vi "Inspect Weight Fiducials.vi"(5 "Dispose Images?":bool, 6 "WorkTable Class in":refnum<class "WorkTable Class.lvclass">=refnum, 7 "Glue Pathways":T7 {"BBM Slot" items=["Slot 1", "Slot 2", "Slot 3", "Slot 4"]; "Weight Slot" items=["Slot 1", "Slot 2", "Slot 3", "Slot 4"]; "Glue Slot" items=["Slot 1", "Slot 2", "Slot 3", "Slot 4"]; "Stamp Slot" items=["Slot 1", "Slot 2", "Slot 3", "Slot 4"]; "HDI Slot" items=["Slot 1", "Slot 2", "Slot 3", "Slot 4"]}, 8 "error in":errorcluster, 9 "Console Log in":refnum<class "Console Log.lvclass">, 10 "Single Path in":T6, 11 "CameraTool in":refnum<class "CameraTool Class.lvclass">) -> (0 "error out":errorcluster, 1 "Console Log out":refnum<class "Console Log.lvclass">, 2 "Single Path out":T6, 3 "CameraTool out":refnum<class "CameraTool Class.lvclass">)   [LabVIEW 2017, in "Gluing Procedure.lvclass"]
uses:
  Gluing Procedure.lvclass
  Shared Components/Config Manager Class/Type Definitions/Named Position.ctl
  Shared Components/CameraTool Class/CameraTool Class.lvclass
  Application Utilities/Console Log/Console Log.lvclass
  UI typedefs/Glue Path.ctl
  Shared Components/WorkTable Class/WorkTable Class.lvclass
  Shared Components/Vec3d Class/Vec3d Class.lvclass
  <vilib>/vision/Image Controls.llb/IMAQ Image.ctl
  Shared Components/Utils/Type Definitions/Physical Image.ctl
  Shared Components/Utils/Type Definitions/Fiducial with Source.ctl
  Shared Components/Utils/Type Definitions/Fiducial Image.ctl
  Shared Components/Utils/Type Definitions/Part Fiducials.ctl
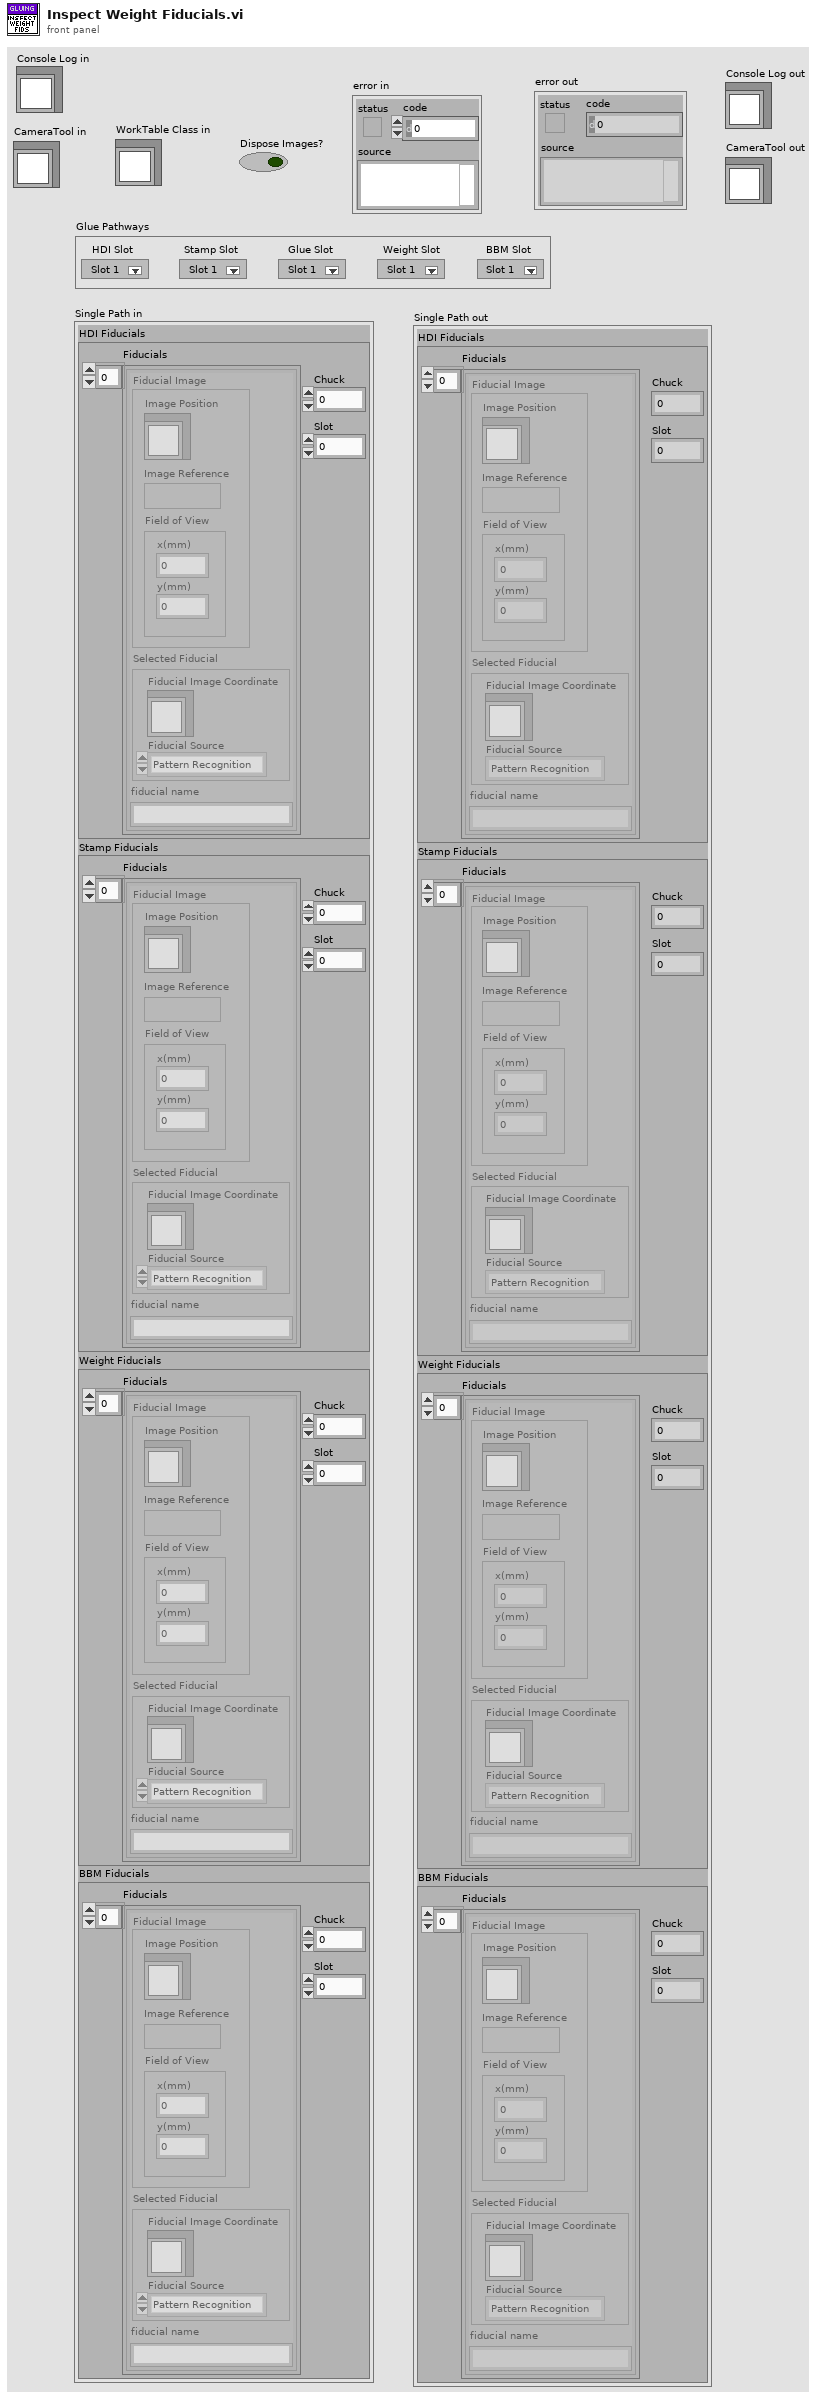
[diagram p1: front panel]
types:
  T1 = typedef "Part Fiducials.ctl" = cluster{"Fiducials":T2[], "Chuck":i32, "Slot":i32}
  T2 = typedef "Fiducial Image.ctl" = cluster{"Fiducial Image":T3, "Selected Fiducial":T5, "fiducial name":string}
  T3 = typedef "Physical Image.ctl" = cluster{"Image Position":refnum<class "Vec3d Class.lvclass">, "Image Reference":T4, "Field of View":cluster{"x(mm)":dbl, "y(mm)":dbl}}
  T4 = typedef "IMAQ Image.ctl" = refnum<image>
  T5 = typedef "Fiducial with Source.ctl" = cluster{"Fiducial Image Coordinate":refnum<class "Vec3d Class.lvclass">, "Fiducial Source":enum16{"Pattern Recognition", "User", "Error", "Default"}}
  T6 = cluster{"HDI Fiducials":T1, "Stamp Fiducials":T1, "Weight Fiducials":T1, "BBM Fiducials":T1}
  T7 = typedef "Glue Path.ctl" = cluster{"HDI Slot ":i32, "Stamp Slot":i32, "Glue Slot":i32, "Weight Slot":i32, "BBM Slot":i32}
  T8 = typedef "Named Position.ctl" = enum16{"home", "module_chuck_0", "module_chuck_1", "module_chuck_2", "module_chuck_3", "module_chuck_4", "glue_reservoir_chuck", "stamp_tool_chuck", "weight_tool_chuck", "needle_calibration", "needle_calibration_camera", "tool_rack_pos_0_in", "tool_rack_pos_0_out", "tool_rack_pos_1_in", "tool_rack_pos_1_out", "tool_rack_pos_2_in", "tool_rack_pos_2_out", "front_load_position", "grabber_start_pos", "between_chuck_0_and_1", "between_chuck_2_and_3"}
  T9 = typedef "Worktable_Weight.ctl" = cluster{"Weight State":enum16{"Empty", "Populated"}, "Weight Type":T10, "Location/Orientation":T11}
  T10 = typedef "Weight Type.ctl" = enum16{"Weight 1", "Weight 2", "Weight 3", "Weight 4", "Weight 5", "Weight 6", "Weight 7", "Weight 8", "Weight 9", "Weight 10", "Weight 11", "Weight 12", "Weight 13", "Weight 14", "Weight 15", "Weight 16"}
  T11 = typedef "Position_Orientation.ctl" = cluster{"Center":refnum<class "Vec3d Class.lvclass">, "Orientation":refnum<class "Orient3d Class.lvclass">}
  T12 = typedef "Part Type.ctl" = enum16{"BBM", "HDI", "BARE HDI", "GLUERESERVOIR", "STAMP_1", "STAMP_2", "STAMP_3", "STAMP_4", "STAMP_5", "STAMP_6", "STAMP_7", "STAMP_8", "WEIGHT_1", "WEIGHT_2", "WEIGHT_3", "WEIGHT_4", "WEIGHT_5", "WEIGHT_6", "WEIGHT_7", "WEIGHT_8", "WEIGHT_9", "WEIGHT_10", "WEIGHT_11", "WEIGHT_12", "WEIGHT_13", "WEIGHT_14", "WEIGHT_15", "WEIGHT_16", "PICKER_TOOL", "GRABER_TOOL", "TFPX_HDI_V2"}
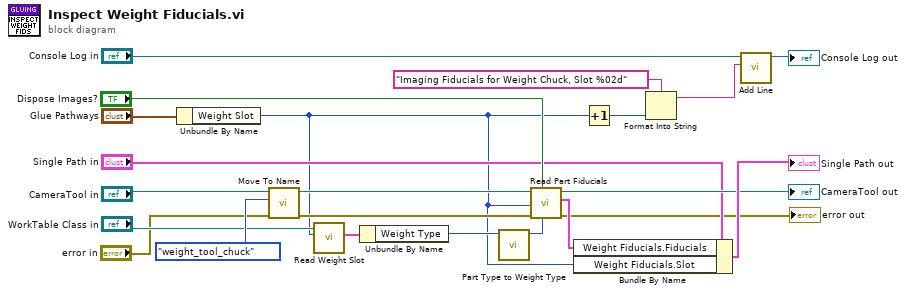
[diagram p0: block diagram]
diagram:
  n1 = Unbundle By Name("Glue Pathways") -> ("Weight Slot"=w1:i32)
  n2 = call-dynamic "Move To Name.vi"("error in"="error in", "Destination"=Named_Position."weight_tool_chuck", "Gantry in"="CameraTool in") -> ("error out"=w8:errorcluster, "Gantry out"=w12:refnum<class "CameraTool Class.lvclass">)  [unwired: 7 in]
  n3 = call "Read Weight Slot.vi"("weight slot"=w1, "WorkTable Class in"="WorkTable Class in") -> ("Weight Slot"=w21:T9)  [unwired: 7 in, 2 out]
  n4 = Unbundle By Name(w21) -> ("Weight Type"=w20:T10)
  n5 = call "Part Type to Weight Type.vi"("Weight Type"=w20) -> ("Part Type"=w18:T12)  [unwired: 9 in, 1 out]
  n6 = call-dynamic "Read Part Fiducials.vi"("Part Type"=w18, "Dispose Images?"="Dispose Images?", "error in"=w8, "Slot"=w1, "CameraTool in"=w12) -> ("error out"=→"error out":errorcluster, "Fiducials"=w17:T2[], "CameraTool out"=→"CameraTool out":refnum<class "CameraTool Class.lvclass">)  [unwired: 4 in]
  n7 = Bundle By Name(cluster="Single Path in", "Weight Fiducials.Fiducials"=w17, "Weight Fiducials.Slot"=w1) -> (→"Single Path out":T6)
  n8 = Increment(x=w1) -> (x+1=w5:i32)
  n9 = Format Into String(format string="Imaging Fiducials for Weight Chuck, Slot %02d", w5) -> (resulting string=w3:string)  [unwired: 2 in, 1 out]
  n10 = call "Add Line.vi"("String"=w3, "Console Log in"="Console Log in") -> ("Console Log out"=→"Console Log out":refnum<class "Console Log.lvclass">)  [unwired: 8 in, 1 out]
